vi "Tell Reply.vi"(4 "Priority":bool, 10 "Msg":refnum<class "Msg.lvclass">, 11 "TEMPLATE Actor in":refnum<class "TEMPLATE Actor.lvclass">) -> (0 "Error out":errorcluster)   [LabVIEW 2025, in "_Template.lvlib" / "Templates.lvlib" / "TEMPLATE Actor.lvlib" / "TEMPLATE Actor.lvclass"]
uses:
  TEMPLATE Actor.lvclass
  jettl/jettl/Msg/Msg.lvclass
  jettl/jettl/Actor/Actor/Actor.lvclass
  TEMPLATE Actor.lvclass/TEMPLATE Actor.ctl
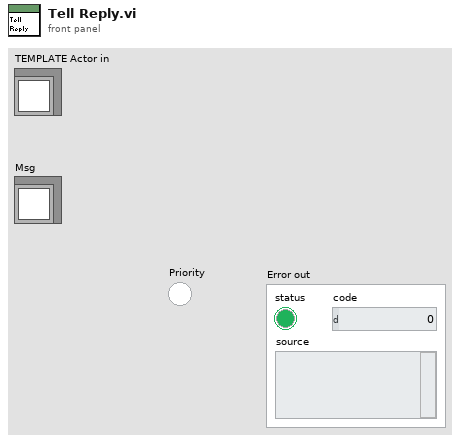
[diagram p1: front panel]
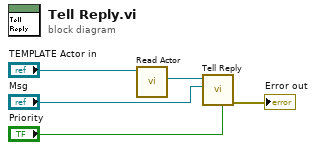
[diagram p0: block diagram]
diagram:
  n1 = call-dynamic "Read Actor.vi"("TEMPLATE Actor in"="TEMPLATE Actor in") -> ("Actor"=w1:refnum<class "Actor.lvclass">)  [unwired: 10 in]
  n2 = call-dynamic "Tell Reply.vi"("Priority"="Priority", "Msg"="Msg", "Actor in"=w1) -> ("Error out"=→"Error out":errorcluster)  [unwired: 8 in]
